vi "Read Transfers.vi"(8 "error in (no error)":errorcluster, 11 "Configuration.Transfer Group in":refnum<class "Configuration.Transfer Group.lvclass">) -> (0 "error out":errorcluster, 2 "Transfers":refnum<class "Configuration.Transfer.lvclass">[](array[class]), 3 "Configuration.Transfer Group out":refnum<class "Configuration.Transfer Group.lvclass">)   [LabVIEW 2016, in "Data Sharing Framework.Configuration.lvlib" / "Configuration.Transfer Group.lvclass"]
uses:
  Configuration.Transfer Group.lvclass
  Configuration.Transfer/Configuration.Transfer.lvclass
  Configuration.Transfer Group.lvclass/Configuration.Transfer Group.ctl
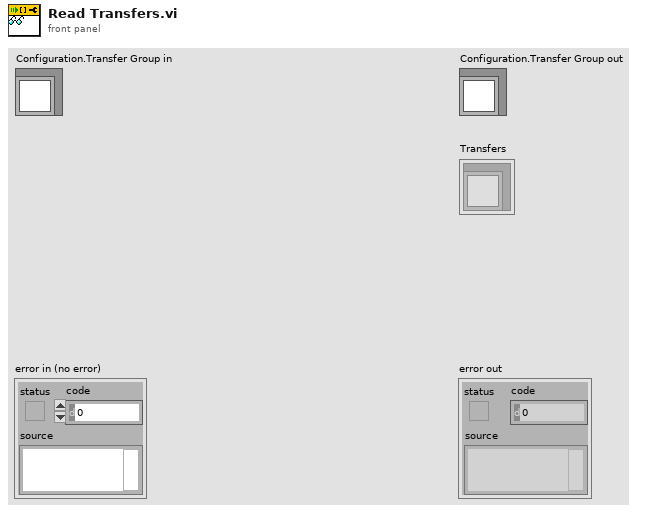
[diagram p1: front panel]
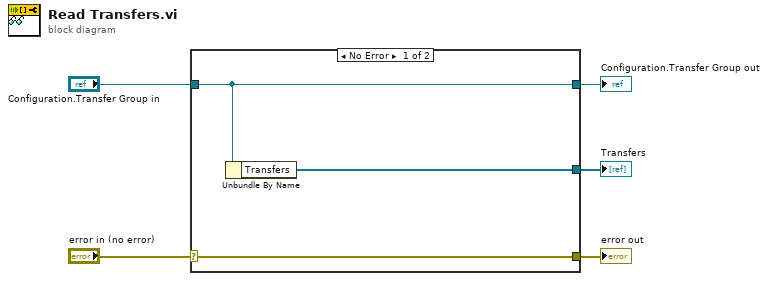
[diagram p0: block diagram]
diagram:
  n1 = case shown="No Error" "error in (no error)" {
    selector: "error in (no error)" -> [w8 w9]
    tunnel: [w8 w9] -> w4
    tunnel: [w7 w10] -> w2
    tunnel: "Configuration.Transfer Group in" -> [w7 w10]
    tunnel: [w6 _] -> w1
    frame No Error {
      n2 = Unbundle By Name(w7) -> ("Transfers"=w6:refnum<class "Configuration.Transfer.lvclass">[])
    }
    frame Error {
    }
  }
  "error out" <- w4
  "Configuration.Transfer Group out" <- w2
  "Transfers" <- w1
